vi "set_motor_diag.vi"(0 "First?":bool, 1 "Voltage Step2":dbl, 2 "Steps":dbl, 5 "Initial Voltage (V)":dbl, 7 "Final Voltage (V) 2":dbl, 9 "Voltage Step (V)":dbl, 11 "Final Voltage (V)":dbl, 12 "error in (no error)":errorcluster, 13 "Physical Channel":tag="Dev1/ao0") -> (4 "Next Voltage (V)":dbl, 10 "Last Step?":bool, 15 "error out":errorcluster)   [LabVIEW 2013]
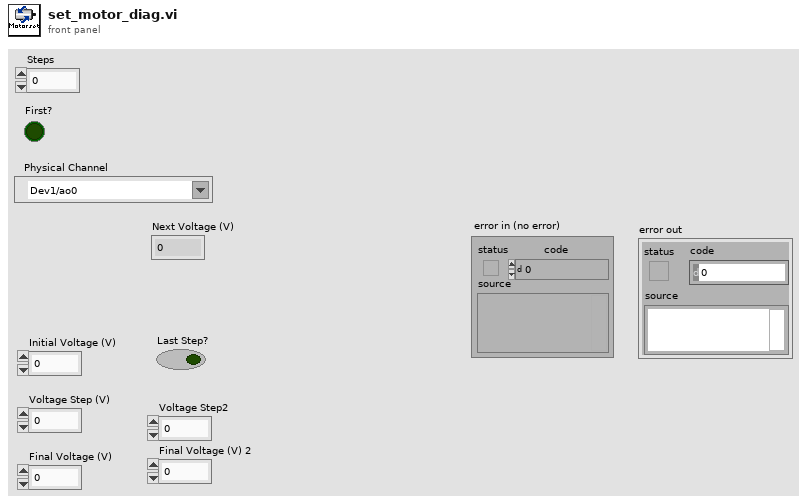
[diagram p1: front panel]
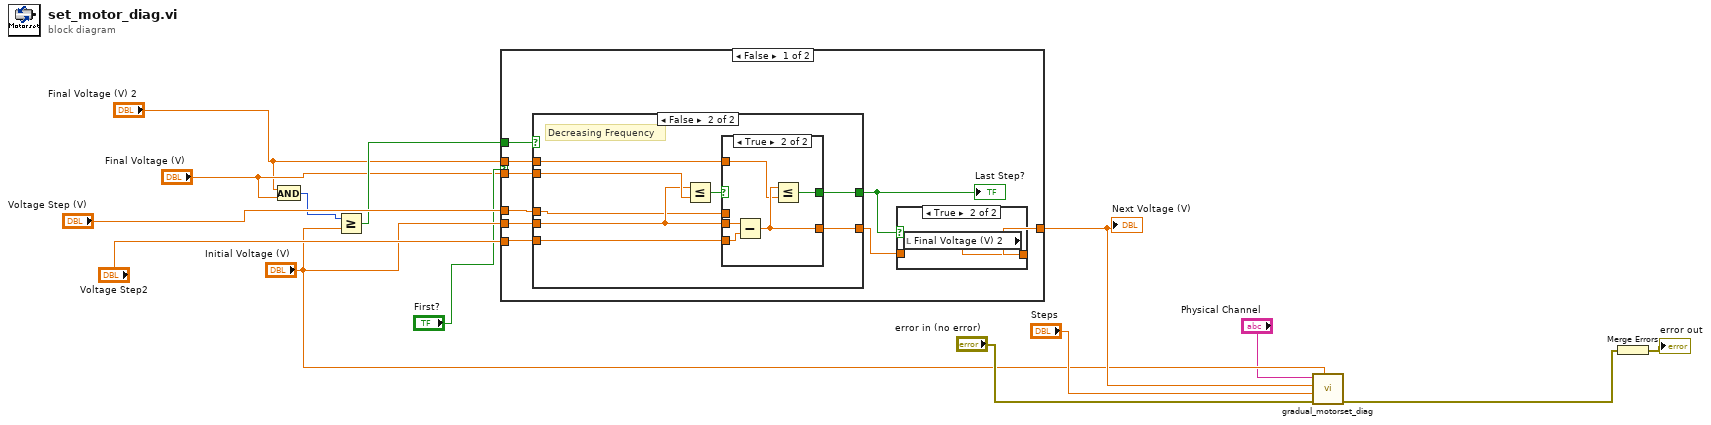
[diagram p0: block diagram]
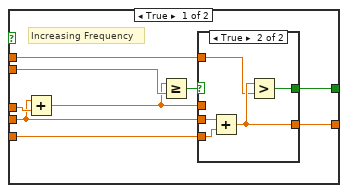
[diagram p3: hidden frame]
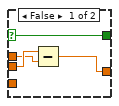
[diagram p5: hidden frame]
diagram:
  n1 = And(x="Final Voltage (V) 2", y="Final Voltage (V)") -> (x .and. y?=w2:i32)
  n2 = Greater Or Equal?(x=w2, y="Initial Voltage (V)") -> (x >= y?=w13:bool)
  n3 = case shown="False" "First?" {
    tunnel: "Voltage Step (V)" -> [w23 _]
    tunnel: w13 -> [w22 _]
    tunnel: "Voltage Step2" -> [w21 _]
    tunnel: [w15 w59] -> w9
    tunnel: "Initial Voltage (V)" -> [w20 w59]
    tunnel: "Final Voltage (V)" -> [w19 _]
    tunnel: "Final Voltage (V) 2" -> [w18 _]
    frame False {
      n4 = case shown="False" w22 {
        tunnel: w23 -> [w33 w42]
        tunnel: w19 -> [w34 w49]
        tunnel: [w31 w46] -> w17
        tunnel: [w29 w47] -> w16
        tunnel: w20 -> [w26 w43]
        tunnel: w21 -> [w28 w45]
        tunnel: w18 -> [w27 w44]
        frame True {
          # "Increasing Frequency"
          n5 = Add(x=w26, y=w33) -> (x+y=w30:dbl)
          n6 = Greater Or Equal?(x=w30, y=w34) -> (x >= y?=w32:bool)
          n7 = case shown="True" w32 {
            selector: w32 -> [w36 _]
            tunnel: [w36 w41] -> w31
            tunnel: w30 -> [w35 _]
            tunnel: [w35 w40] -> w29
            tunnel: w28 -> [_ w39]
            tunnel: w27 -> [_ w38]
            tunnel: w26 -> [_ w37]
            frame False {
            }
            frame True {
              n8 = Add(x=w37, y=w39) -> (x+y=w40:dbl)
              n9 = Greater?(x=w40, y=w38) -> (0:w41:bool)
            }
          }
        }
        frame False {
          # "Decreasing Frequency"
          n10 = Less Or Equal?(x=w43, y=w49) -> (x <= y?=w48:bool)
          n11 = case shown="True" w48 {
            selector: w48 -> [w53 _]
            tunnel: [w53 w57] -> w46
            tunnel: w43 -> [w52 w58]
            tunnel: [w50 w56] -> w47
            tunnel: w45 -> [_ w55]
            tunnel: w44 -> [_ w54]
            tunnel: w42 -> [w51 _]
            frame False {
              n12 = Subtract(x=w52, y=w51) -> (x-y=w50:dbl)
            }
            frame True {
              n13 = Subtract(x=w58, y=w55) -> (x-y=w56:dbl)
              n14 = Less Or Equal?(x=w56, y=w54) -> (x <= y?=w57:bool)
            }
          }
        }
      }
      "Last Step?" <- w17
      n15 = case shown="True" w17 {
        tunnel: w16 -> [w24 _]
        tunnel: [w24 w25] -> w15
        frame False {
        }
        frame True {
          n16 = local read "Final Voltage (V) 2"() -> (w25:dbl)
        }
      }
    }
    frame True {
    }
  }
  "Next Voltage (V)" <- w9
  n17 = call "gradual_motorset_diag.vi"("Initial Voltage (V)"="Initial Voltage (V)", "error in (no error)"="error in (no error)", "Steps"="Steps", "Next Voltage (V)"=w9, "Physical Channel"="Physical Channel") -> ("error out"=w6:errorcluster)  [unwired: 6 in]
  n18 = Merge Errors(w6) -> (→"error out":errorcluster)
